vi "rad_Deploy Images with Progress.vi"(6 "Deployment Notifiers":T1[](array[typedef]), 7 "temp folder":path, 8 "error in (no error)":errorcluster, 9 "Target Config Options in":T4={"NumInBatch"=0, "Target Config Operation"=enum."No Config", "Target Name"="", "Increment Static IPs"=FALSE, "Change Target Name"=FALSE, "Primary NIC"={"MAC address"="", "IP Address Request Mode"=2, "IP address"="", "Subnet mask"="", "Gateway"="", "DNS server"=""}} {"Primary NIC"."IP Address Request Mode" items=["Static"=1, "DHCP/Link-Local"=2, "Link-Local Only"=4, "DHCP Only"=8]}, 10 "RT Deployment Targets in":T2[](array[typedef]) {"Primary NIC"."IP Address Request Mode" items=["Static"=1, "DHCP/Link-Local"=2, "Link-Local Only"=4, "DHCP Only"=8]}, 11 "image path":path) -> (0 "error out":errorcluster, 1 "Target Config Options out":T4={"NumInBatch"=0, "Target Config Operation"=enum."No Config", "Target Name"="", "Increment Static IPs"=FALSE, "Change Target Name"=FALSE, "Primary NIC"={"MAC address"="", "IP Address Request Mode"=2, "IP address"="", "Subnet mask"="", "Gateway"="", "DNS server"=""}} {"Primary NIC"."IP Address Request Mode" items=["Static"=1, "DHCP/Link-Local"=2, "Link-Local Only"=4, "DHCP Only"=8]}, 2 "Error Occurred":bool[](array[boolean]))   [LabVIEW 2013]
uses:
  TypeDefs/rad_Target Configuration Settings.ctl
  TypeDefs/rad_Target Configuration Operations.ctl
  Targets/TypeDefs/rad_Target Network Settings.ctl
  Targets/TypeDefs/rad_Target Information.ctl
  TypeDefs/rad_Application Image Properties.ctl
  TypeDefs/rad_FPGA Properties.ctl
  TypeDefs/rad_FPGA Flash Properties.ctl
  TypeDefs/rad_Deployment Notifiers.ctl
  TypeDefs/rad_Deployment Status Data Type.ctl
  TypeDefs/rad_Deployment Progress Data Type.ctl
  Targets/TypeDefs/rad_Initialize Access Types.ctl
  <vilib>/nisyscfg/Close (System).vi
  <vilib>/nisyscfg/Set System Image (Folder).vi
  <vilib>/nisyscfg/nisyscfg.lvlib
panel:
  in  "State Variables":T10={"INI Modified"=FALSE, "Target Config. Options"={"NumInBatch"=0, "Target Config Operation"=enum."No Config", "Target Name"="", "Increment Static IPs"=FALSE, "Change Target Name"=FALSE, "Primary NIC"={"MAC address"="", "IP Address Request Mode"=2, "IP address"="", "Subnet mask"="", "Gateway"="", "DNS server"=""}}, "RT Deployment Targets"=[], "AppImage Properties"={"Name"="", "Version"="", "Time"=timestamp(0 s since 1904-01-01), "Description"="", "Key"="", "Chassis"="", "FPGA Properties"=[], "Model"="", "Retrieve"=[], "Deploy"=[], "Installed Software"=[]}, "Deployment Notifiers"=[], "Post-deployment access"=enum."Admin unless unlocked"} {"RT Deployment Targets"."Primary NIC"."IP Address Request Mode" items=["Static"=1, "DHCP/Link-Local"=2, "Link-Local Only"=4, "DHCP Only"=8]; "Target Config. Options"."Primary NIC"."IP Address Request Mode" items=["Static"=1, "DHCP/Link-Local"=2, "Link-Local Only"=4, "DHCP Only"=8]}
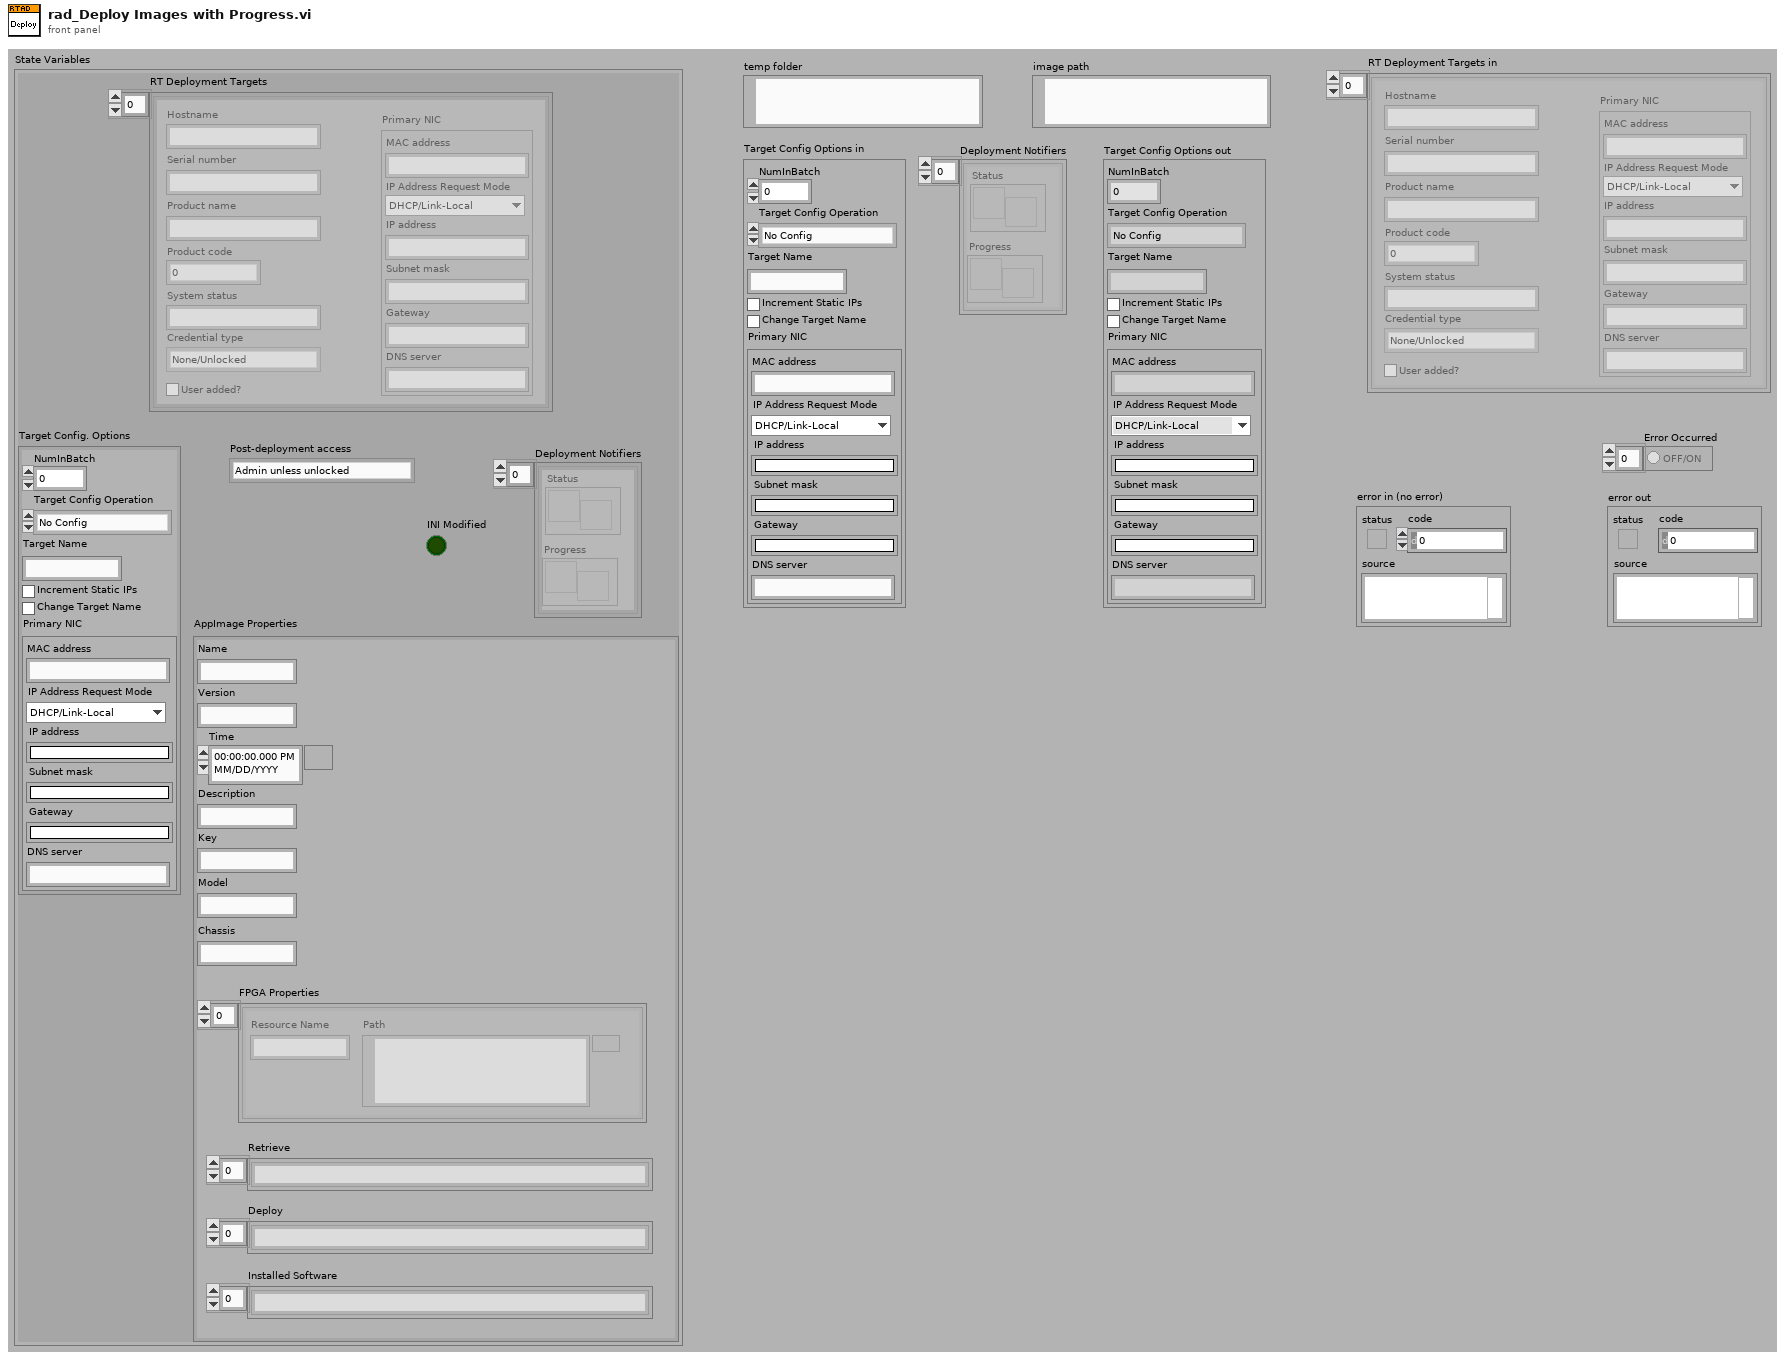
[diagram p1: front panel]
types:
  T1 = typedef "rad_Deployment Notifiers.ctl" = cluster{"Status":refnum<notifier>, "Progress":refnum<notifier>}
  T2 = typedef "rad_Target Information.ctl" = cluster{"Hostname":string, "Serial number":string, "Product name":string, "Product code":i32, "System status":string, "Credential type":enum16{"None/Unlocked", "FTP Password", "NIAuth Credentials"}, "User added?":bool, "Primary NIC":T3}
  T3 = typedef "rad_Target Network Settings.ctl" = cluster{"MAC address":string, "IP Address Request Mode":i32, "IP address":string, "Subnet mask":string, "Gateway":string, "DNS server":string}
  T4 = typedef "rad_Target Configuration Settings.ctl" = cluster{"NumInBatch":u32, "Target Config Operation":T5, "Target Name":string, "Increment Static IPs":bool, "Change Target Name":bool, "Primary NIC":T3}
  T5 = typedef "rad_Target Configuration Operations.ctl" = enum8{"No Config", "Image Config", "Static Config"}
  T6 = typedef "rad_Application Image Properties.ctl" = cluster{"Name":string, "Version":string, "Time":timestamp, "Description":string, "Key":string, "Chassis":string, "FPGA Properties":T7, "Model":string, "Retrieve":string[], "Deploy":string[], "Installed Software":string[]}
  T7 = typedef "rad_FPGA Properties.ctl" = T8[]
  T8 = typedef "rad_FPGA Flash Properties.ctl" = cluster{"Resource Name":string, "Path":path}
  T9 = typedef "rad_Initialize Access Types.ctl" = enum16{"Anonymous read-only", "Admin unless unlocked", "Admin always"}
  T10 = cluster{"INI Modified":bool, "Target Config. Options":T4, "RT Deployment Targets":T2[], "AppImage Properties":T6, "Deployment Notifiers":T1[], "Post-deployment access":T9}
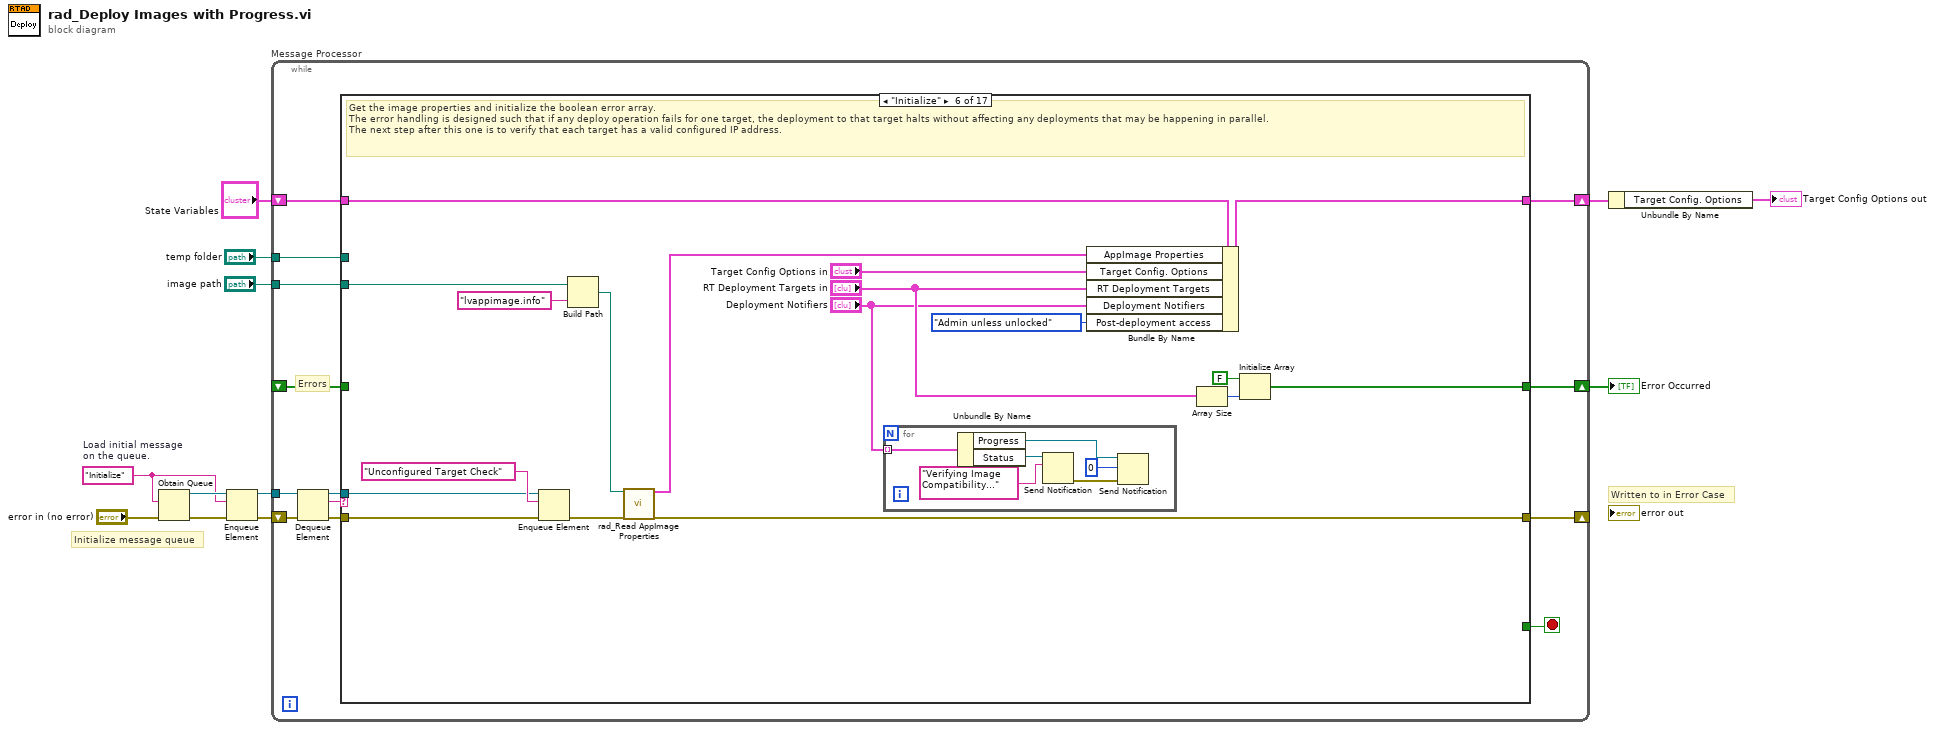
[diagram p0: block diagram]
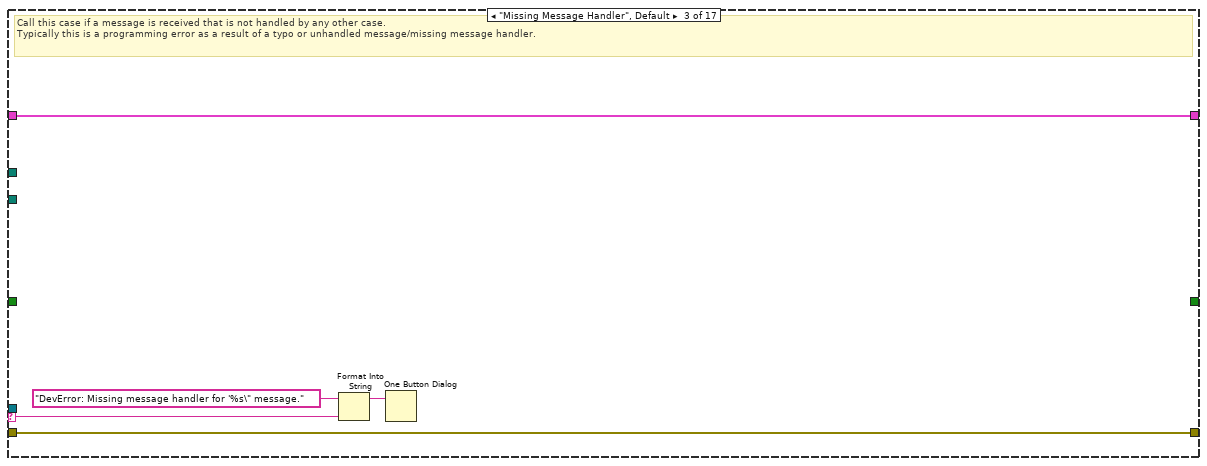
[diagram p4: hidden frame]
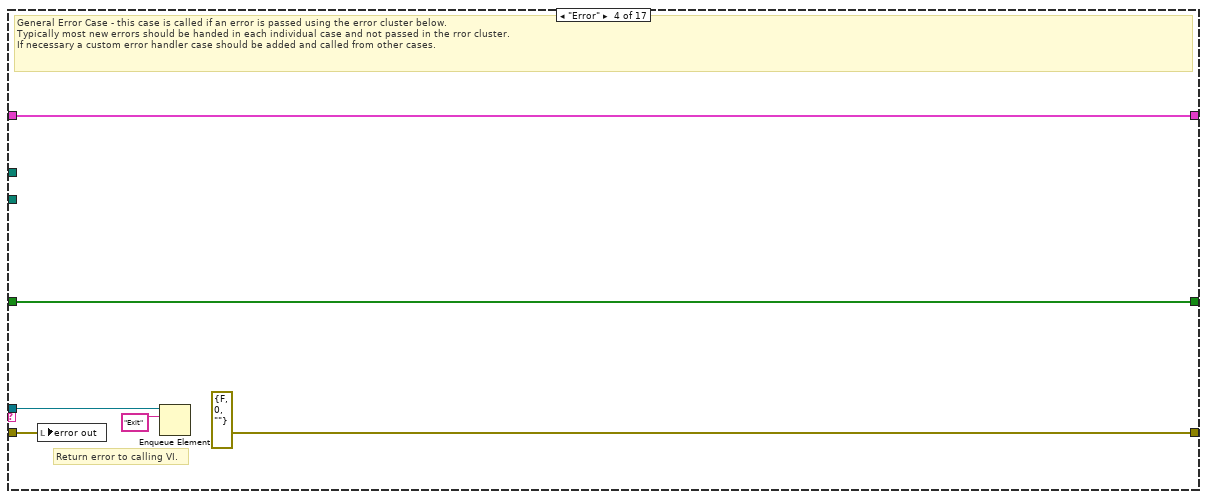
[diagram p5: hidden frame]
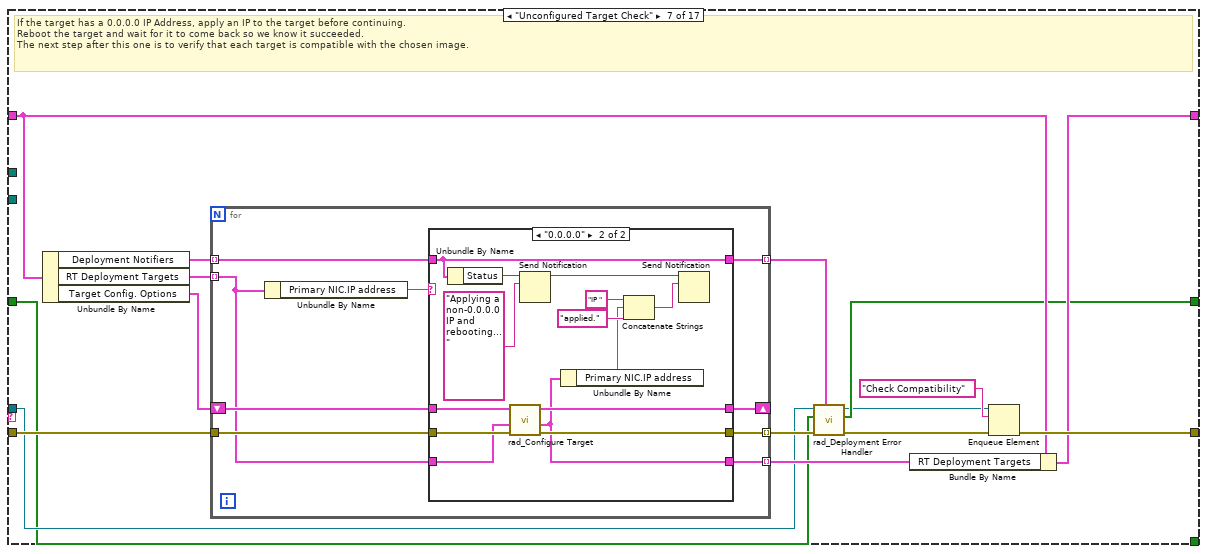
[diagram p7: hidden frame]
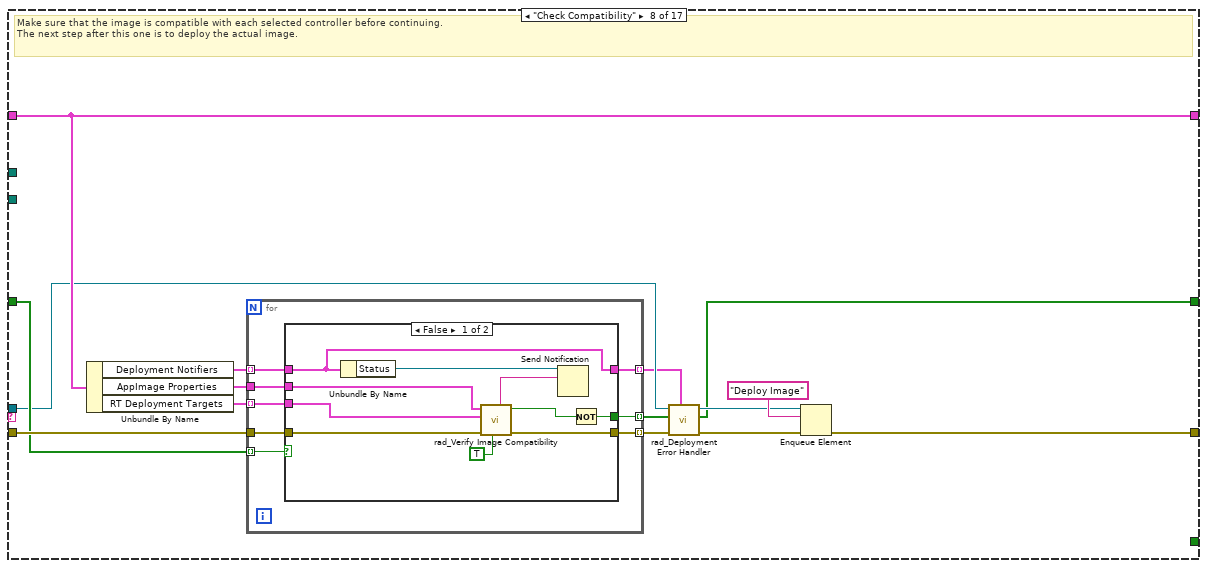
[diagram p9: hidden frame]
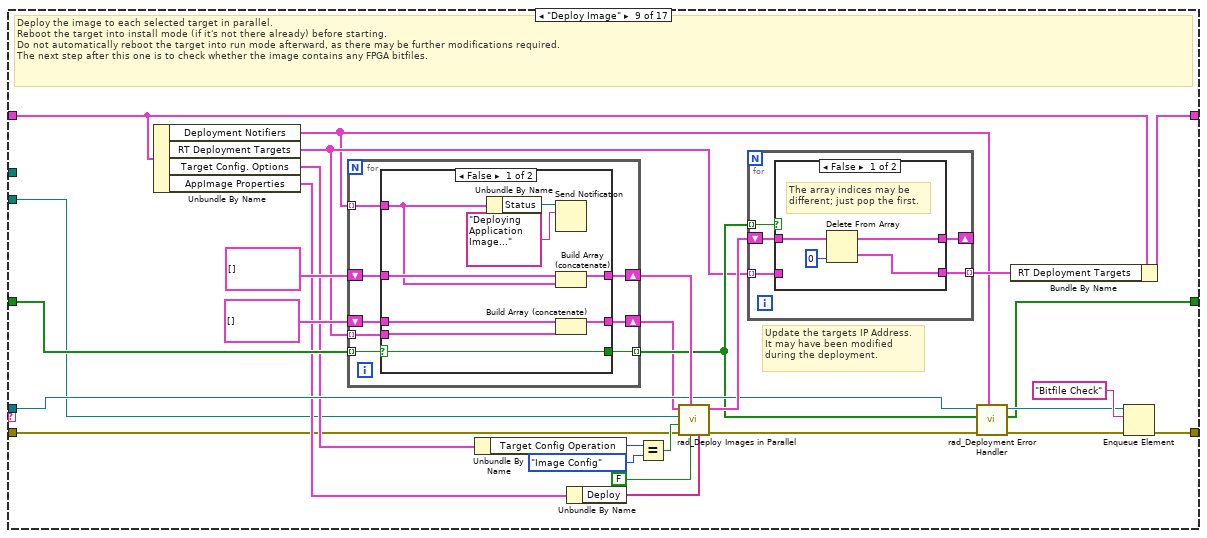
[diagram p11: hidden frame]
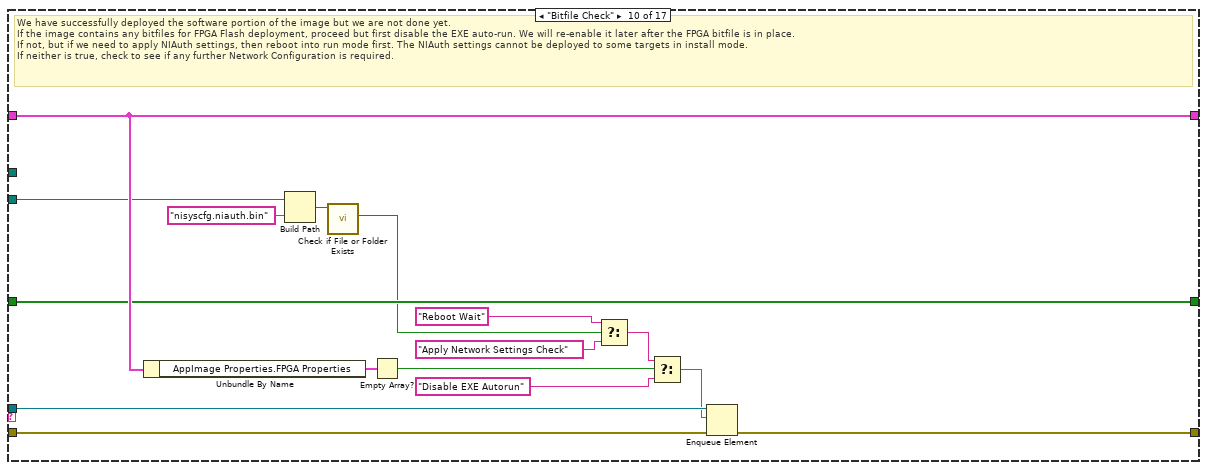
[diagram p14: hidden frame]
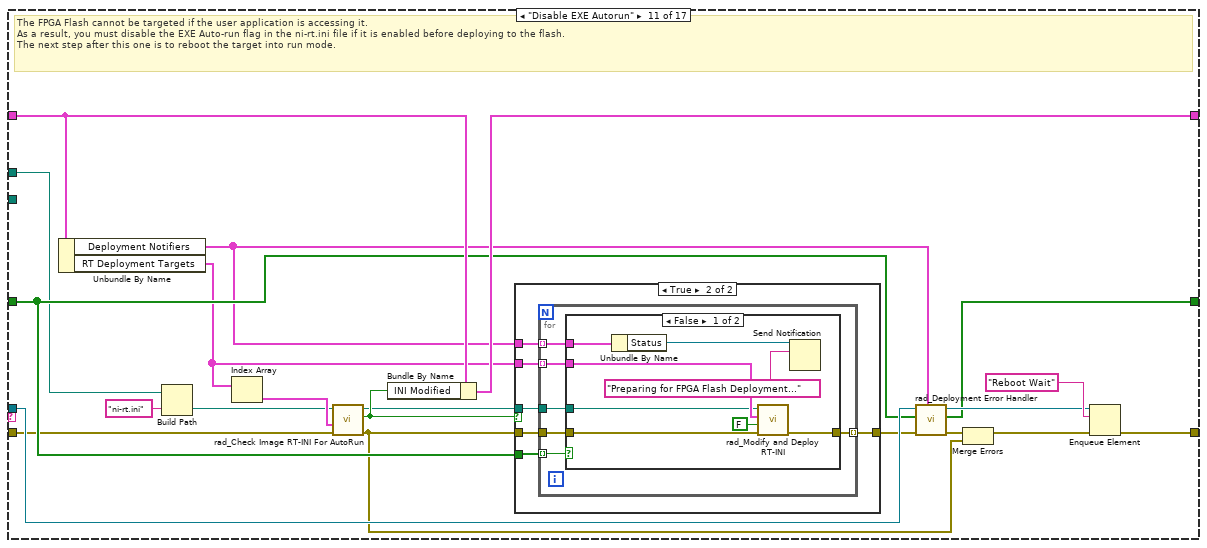
[diagram p15: hidden frame]
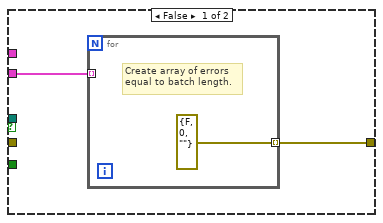
[diagram p16: hidden frame]
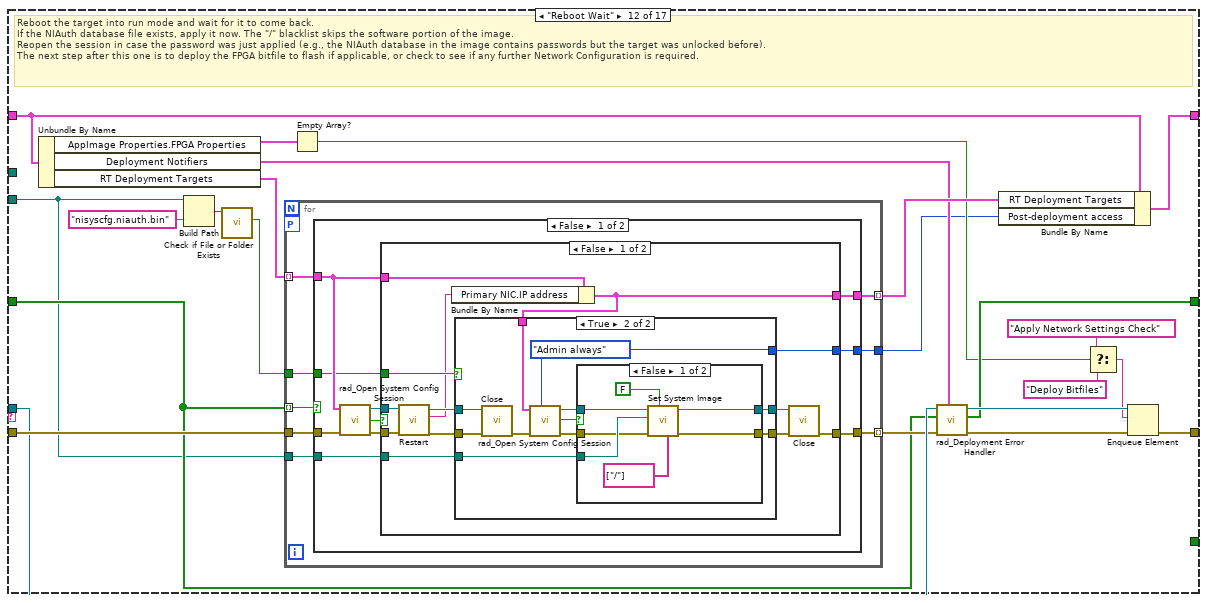
[diagram p18: hidden frame]
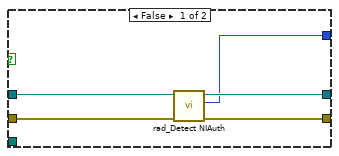
[diagram p19: hidden frame]
diagram:
  w1 = "Initialize"  # Load initial message on the queue.
  # "Written to in Error Case"
  # "Initialize message queue"
  n1 = Obtain Queue(element data type=w1, error in (no error)="error in (no error)") -> (queue out=w12:refnum<queue>, error out=w3:errorcluster)  [unwired: 3 in, 1 out]
  n2 = Enqueue Element(queue=w12, element=w1, error in (no error)=w3) -> (queue out=w4:refnum<queue>, error out=w2:errorcluster)  [unwired: 1 in, 1 out]
  n3 = while "Message Processor" {
    shift-left: w2 -> [w21]
    shift-right: [w14] -> _
    tunnel: w4 -> [w22]
    shift-left: "State Variables" -> [w25]
    shift-right: [w24] -> w9
    tunnel: "temp folder" -> [w18]
    tunnel: "image path" -> [w17]
    shift-right: [w15] -> w5
    shift-left: _ -> [w16]
    stop <- w13 stop-if-true
    # "Errors"
    n4 = Dequeue Element(queue=w22, error in (no error)=w21) -> (queue out=w23:refnum<queue>, element=w19:string, error out=w20:errorcluster)  [unwired: 1 in, 1 out]
    n5 = case shown="\"Initialize\"" w19 {
      selector: w19 -> [_ _ w33 _ _ _ _ _ _ _ _ _ _ _ _ _ _]
      tunnel: [w27 w30 w35 w41 w43 w60 w80 w124 w166 w219 w239 w284 w372 w412 w441 w488 w512] -> w24
      tunnel: w25 -> [w27 w30 w35 w41 w43 w61 w79 w124 w167 w219 w240 w286 w372 w412 w439 w488 w512]
      tunnel: w23 -> [_ _ _ w40 _ w45 w70 w117 w164 w220 w238 w282 w366 w409 w432 w495 w514]
      tunnel: w20 -> [w26 w29 w34 w37 w42 w50 w83 w119 w147 w218 w224 w287 w355 w400 w440 w497 w515]
      tunnel: [w26 w29 w34 errorcluster {"status"=FALSE, "code"=0, "source"=""} ("error out") w42 w51 w82 w125 w174 w221 w242 w289 w373 w411 w445 w499 w513] -> w14
      tunnel: w18 -> [_ _ _ _ _ _ _ _ _ _ w225 _ _ w401 _ _ _]
      tunnel: w17 -> [_ _ _ _ _ w49 _ _ w148 w213 _ w272 w354 _ _ _ _]
      tunnel: [_ w28 _ w36 _ w56 w74 w112 w159 w217 w235 w280 w365 w407 w430 w493 w510] -> w15
      tunnel: w16 -> [_ w28 _ w36 _ _ w68 w118 w172 w217 w232 w277 w361 w405 w425 w490 w510]
      tunnel: [_ _ _ _ _ _ _ _ _ _ _ _ _ _ _ _ TRUE] -> w13
      frame "---------- Framework Operations ----------" {
        # "Dummy case to add a seperator in the Case Structure menu."
      }
      frame "", "Idle" {
        # "Idle Case - this case is called after a Timeout on the Get Next Message from Queue VI, if no new messages are present on the queue.\nThis case can be used for housekeeping tasks such as updating the UI."
      }
      frame "Missing Message Handler", Default {
        # "Call this case if a message is received that is not handled by any other case.\nTypically this is a programming error as a result of a typo or unhandled message/missing message handler."
        n6 = Format Into String(format string="DevError: Missing message handler for '%s\" message." ("message"), w33) -> (resulting string=w31:string)  [unwired: 2 in, 1 out]
        n7 = One Button Dialog(message=w31) -> ()  [unwired: 2 out]
      }
      frame "Error" {
        # "Return error to calling VI."
        # "General Error Case - this case is called if an error is passed using the error cluster below.\nTypically most new errors should be handed in each individual case and not passed in the rror cluster.\nIf necessary a custom error handler case should be added and called from other cases."
        n8 = local write "error out"(w37) -> ()
        n9 = Enqueue Element(queue=w40, element="Exit") -> ()  [unwired: 2 in, 3 out]
      }
      frame "----------Application Operations ----------" {
        # "Dummy case to add a seperator in the Case Structure menu."
      }
      frame "Initialize" {
        # "Get the image properties and initialize the boolean error array. \nThe error handling is designed such that if any deploy operation fails for one target, the deployment to that target halts without affecting any deployments that may be happening in parallel. \nThe next step after this one is to verify that each target has a valid configured IP address."
        n10 = Enqueue Element(queue=w45, element="Unconfigured Target Check", error in (no error)=w50) -> (error out=w47:errorcluster)  [unwired: 1 in, 2 out]
        n11 = Build Path(base path=w49, name or relative path="lvappimage.info") -> (appended path=w52:path)
        n12 = call "rad_Read AppImage Properties.vi"("AppImage Properties Path"=w52, "error in (no error)"=w47) -> ("AppImage Properties"=w48:T6, "error out"=w51:errorcluster)  [unwired: 12 in, 4 out]
        n13 = for {
          tunnel: "Deployment Notifiers" -> [w66] mode=indexing
          n14 = Unbundle By Name(w66) -> ("Progress"=w64:refnum<notifier>, "Status"=w65:refnum<notifier>)
          n15 = Send Notification(notification="Verifying Image Compatibility...", notifier=w65) -> (error out=w63:errorcluster)  [unwired: 1 in, 1 out]
          n16 = Send Notification(notification=0, notifier=w64, error in (no error)=w63) -> ()  [unwired: 2 out]
        }
        n17 = Bundle By Name(cluster=w61, "AppImage Properties"=w48, "Target Config. Options"="Target Config Options in", "RT Deployment Targets"="RT Deployment Targets in", "Deployment Notifiers"="Deployment Notifiers", "Post-deployment access"=rad_Initialize_Access_Types."Admin unless unlocked") -> (w60:T10)
        n18 = Array Size(array="RT Deployment Targets in") -> (size(s)=w57:i32)
        n19 = Initialize Array(FALSE, w57) -> (w56:bool[])
      }
      frame "Unconfigured Target Check" {
        # "If the target has a 0.0.0.0 IP Address, apply an IP to the target before continuing. \nReboot the target and wait for it to come back so we know it succeeded. \nThe next step after this one is to verify that each target is compatible with the chosen image."
        n20 = Unbundle By Name(w79) -> ("Deployment Notifiers"=w78:T1[], "RT Deployment Targets"=w77:T2[], "Target Config. Options"=w76:T4)
        n21 = for {
          tunnel: w83 -> [w90]
          tunnel: [w92] -> w73 mode=indexing
          tunnel: w78 -> [w88] mode=indexing
          tunnel: w77 -> [w87] mode=indexing
          shift-right: [w89] -> _
          shift-left: w76 -> [w91]
          tunnel: [w86] -> w75 mode=indexing
          tunnel: [w85] -> w71 mode=indexing
          n22 = Unbundle By Name(w87) -> ("Primary NIC.IP address"=w84:string)
          n23 = case shown="\"0.0.0.0\"" w84 {
            tunnel: [w96 w102] -> w92
            tunnel: w91 -> [w94 w110]
            tunnel: w90 -> [w96 w103]
            tunnel: [w94 w109] -> w89
            tunnel: w88 -> [w93 w100]
            tunnel: w87 -> [w95 w99]
            tunnel: [w95 w98] -> w86
            tunnel: [w93 w100] -> w85
            frame Default {
            }
            frame "0.0.0.0" {
              n24 = Unbundle By Name(w100) -> ("Status"=w101:refnum<notifier>)
              n25 = call "rad_Configure Target.vi"("error in (no error)"=w103, "Target settings in"=w99, "Target Config Options in"=w110) -> ("error out"=w102:errorcluster, "Target settings out"=w98:T2, "Target Config Options out"=w109:T4)  [unwired: 6 in]
              n26 = Send Notification(notification="Applying a non-0.0.0.0 IP and rebooting...", notifier=w101) -> (notifier out=w107:refnum<notifier>)  [unwired: 1 in, 1 out]
              n27 = Unbundle By Name(w98) -> ("Primary NIC.IP address"=w97:string)
              n28 = Concatenate Strings("IP " ("notification"), w97, "applied." ("string")) -> (w104:string)
              n29 = Send Notification(notification=w104, notifier=w107) -> ()  [unwired: 1 in, 2 out]
            }
          }
        }
        n30 = call "rad_Deployment Error Handler.vi"("Deployment Notifiers"=w71, "error in (no error)"=w73, "Error Occurred"=w68, "Queue in"=w70) -> ("error out"=w72:errorcluster, "Error Occurred"=w74:bool[], "Queue out"=w69:refnum<queue>)  [unwired: 5 in]
        n31 = Bundle By Name(cluster=w79, "RT Deployment Targets"=w75) -> (w80:T10)
        n32 = Enqueue Element(queue=w69, element="Check Compatibility" ("Message Name"), error in (no error)=w72) -> (error out=w82:errorcluster)  [unwired: 1 in, 2 out]
      }
      frame "Check Compatibility" {
        # "Make sure that the image is compatible with each selected controller before continuing.\nThe next step after this one is to deploy the actual image."
        n33 = Unbundle By Name(w124) -> ("Deployment Notifiers"=w121:T1[], "AppImage Properties"=w120:T6, "RT Deployment Targets"=w122:T2[])
        n34 = for {
          tunnel: w122 -> [w131] mode=indexing
          tunnel: w121 -> [w129] mode=indexing
          tunnel: w120 -> [w133]
          tunnel: w119 -> [w132]
          tunnel: w118 -> [w130] mode=indexing
          tunnel: [w128] -> w115 mode=indexing
          tunnel: [w127] -> w116 mode=indexing
          tunnel: [w126] -> w114 mode=indexing
          n35 = case shown="False" w130 {
            selector: w130 -> [_ w146]
            tunnel: w133 -> [w143 _]
            tunnel: w132 -> [w142 w145]
            tunnel: w131 -> [w134 _]
            tunnel: w129 -> [w136 w144]
            tunnel: [w138 w146] -> w128
            tunnel: [w140 w145] -> w127
            tunnel: [w136 w144] -> w126
            frame False {
              n36 = Unbundle By Name(w136) -> ("Status"=w137:refnum<notifier>)
              n37 = call "rad_Verify Image Compatibility.vi"("Require Identical Chassis?"=TRUE, "error in (no error)"=w142, "Target address"=w134, "AppImage Properties"=w143) -> ("error out"=w140:errorcluster, "Compatible?"=w139:bool, "Status message"=w135:string)  [unwired: 5 in]
              n38 = Send Notification(notification=w135, notifier=w137) -> ()  [unwired: 1 in, 2 out]
              n39 = Not(x=w139) -> (.not. x?=w138:bool)
            }
            frame True {
            }
          }
        }
        n40 = call "rad_Deployment Error Handler.vi"("Deployment Notifiers"=w114, "error in (no error)"=w116, "Error Occurred"=w115, "Queue in"=w117) -> ("error out"=w111:errorcluster, "Error Occurred"=w112:bool[], "Queue out"=w113:refnum<queue>)  [unwired: 5 in]
        n41 = Enqueue Element(queue=w113, element="Deploy Image" ("t"), error in (no error)=w111) -> (error out=w125:errorcluster)  [unwired: 1 in, 2 out]
      }
      frame "Deploy Image" {
        # "Update the targets IP Address.\nIt may have been modified\nduring the deployment."
        # "Deploy the image to each selected target in parallel. \nReboot the target into install mode (if it's not there already) before starting.\nDo not automatically reboot the target into run mode afterward, as there may be further modifications required. \nThe next step after this one is to check whether the image contains any FPGA bitfiles."
        n42 = Unbundle By Name(w167) -> ("Deployment Notifiers"=w156:T1[], "RT Deployment Targets"=w157:T2[], "Target Config. Options"=w152:T4, "AppImage Properties"=w151:T6)
        n43 = for {
          tunnel: w156 -> [w192] mode=indexing
          tunnel: w172 -> [w193] mode=indexing
          tunnel: [w191] -> w162 mode=indexing
          tunnel: w157 -> [w190] mode=indexing
          shift-right: [w189] -> w169
          shift-left: T1[] [] ("Deployment Notifiers") -> [w188]
          shift-right: [w187] -> w149
          shift-left: T2[] [] -> [w186]
          n44 = case shown="False" w193 {
            selector: w193 -> [w201 w205]
            tunnel: w192 -> [w196 _]
            tunnel: [w201 w205] -> w191
            tunnel: w190 -> [w194 _]
            tunnel: [w200 w203] -> w189
            tunnel: w188 -> [w199 w203]
            tunnel: [w198 w204] -> w187
            tunnel: w186 -> [w197 w204]
            frame False {
              n45 = Unbundle By Name(w196) -> ("Status"=w195:refnum<notifier>)
              n46 = Send Notification(notification="Deploying Application Image...", notifier=w195) -> ()  [unwired: 1 in, 2 out]
              n47 = Build Array (concatenate)(w199, w196) -> (w200:T1[])
              n48 = Build Array (concatenate)(w197, w194) -> (w198:T2[])
            }
            frame True {
            }
          }
        }
        n49 = Unbundle By Name(w152) -> ("Target Config Operation"=w155:T5)
        n50 = Unbundle By Name(w151) -> ("Deploy"=w150:string[])
        n51 = Equal?(x=w155, y=rad_Target_Configuration_Operations."Image Config" ("x")) -> (x = y?=w153:bool)
        n52 = call "rad_Deploy Images in Parallel.vi"("Deploy"=w150, "restart after imaging (T)"=FALSE ("restart after imaging? (T)"), "Deployment Notifiers"=w169, "error in (no error)"=w147, "apply primary NIC from image (F)"=w153, "image file path in"=w148, "Target addresses in"=w149) -> ("Errors Out"=w163:errorcluster[], "Target addresses out"=w168:T2[])  [unwired: 2 in, 1 out]
        n53 = for {
          tunnel: w162 -> [w179] mode=indexing
          tunnel: w157 -> [w177] mode=indexing
          shift-right: [w175] -> _
          shift-left: w168 -> [w178]
          tunnel: [w176] -> w165 mode=indexing
          n54 = case shown="False" w179 {
            tunnel: w178 -> [w183 w185]
            tunnel: w177 -> [_ w184]
            tunnel: [w181 w184] -> w176
            tunnel: [w182 w185] -> w175
            frame False {
              # "The array indices may be\ndifferent; just pop the first."
              n55 = Delete From Array(array=w183, index=0) -> (deleted portion=w181:T2, array with subset deleted=w182:T2[])  [unwired: 1 in]
            }
            frame True {
              # "An error happened earlier,\nso keep the existing address."
            }
          }
        }
        n56 = call "rad_Deployment Error Handler.vi"("Deployment Notifiers"=w156, "error in (no error)"=w163, "Error Occurred"=w162, "Queue in"=w164) -> ("error out"=w160:errorcluster, "Error Occurred"=w159:bool[], "Queue out"=w161:refnum<queue>)  [unwired: 5 in]
        n57 = Bundle By Name(cluster=w167, "RT Deployment Targets"=w165) -> (w166:T10)
        n58 = Enqueue Element(queue=w161, element="Bitfile Check" ("Message Name"), error in (no error)=w160) -> (error out=w174:errorcluster)  [unwired: 1 in, 2 out]
      }
      frame "Bitfile Check" {
        # "We have successfully deployed the software portion of the image but we are not done yet.\nIf the image contains any bitfiles for FPGA Flash deployment, proceed but first disable the EXE auto-run. We will re-enable it later after the FPGA bitfile is in place.\nIf not, but if we need to apply NIAuth settings, then reboot into run mode first. The NIAuth settings cannot be deployed to some targets in install mode.\nIf neither is true, check to see if any further Network Configuration is required."
        n59 = Unbundle By Name(w219) -> ("AppImage Properties.FPGA Properties"=w216:T7)
        n60 = Build Path(base path=w213, name or relative path="nisyscfg.niauth.bin") -> (appended path=w211:path)
        n61 = call <vilib>:"Check if File or Folder Exists.vi"("path"=w211) -> ("file or folder exists?"=w208:bool)  [unwired: 8 in, 2 out]
        n62 = Empty Array?(array=w216) -> (empty?=w214:bool)
        n63 = Select(t="Reboot Wait" ("Title"), s=w208, f="Apply Network Settings Check" ("Title")) -> (s? t:f=w209:string)
        n64 = Select(t=w209, s=w214, f="Disable EXE Autorun" ("Title")) -> (s? t:f=w210:string)
        n65 = Enqueue Element(queue=w220, element=w210, error in (no error)=w218) -> (error out=w221:errorcluster)  [unwired: 1 in, 2 out]
      }
      frame "Disable EXE Autorun" {
        # "The FPGA Flash cannot be targeted if the user application is accessing it.\nAs a result, you must disable the EXE Auto-run flag in the ni-rt.ini file if it is enabled before deploying to the flash.\nThe next step after this one is to reboot the target into run mode."
        n66 = Unbundle By Name(w240) -> ("Deployment Notifiers"=w231:T1[], "RT Deployment Targets"=w230:T2[])
        n67 = Build Path(base path=w225, name or relative path="ni-rt.ini") -> (appended path=w223:path)
        n68 = Index Array(array=w230) -> (element=w226:T2)  [unwired: 1 in]
        n69 = call "rad_Check Image RT-INI For AutoRun.vi"("error in (no error)"=w224, "target settings"=w226, "temp folder"=w223) -> ("error out"=w229:errorcluster, "Run at Startup?"=w228:bool, "temp folder out"=w227:path)  [unwired: 6 in]
        n70 = Bundle By Name(cluster=w240, "INI Modified"=w228) -> (w239:T10)
        n71 = case shown="True" w228 {
          tunnel: [w243 w250] -> w236
          tunnel: w229 -> [_ w251]
          tunnel: w230 -> [w244 w249]
          tunnel: w232 -> [_ w248]
          tunnel: w231 -> [_ w247]
          tunnel: w227 -> [_ w246]
          frame False {
            n72 = for {
              tunnel: w244 -> [_] mode=indexing
              tunnel: [errorcluster {"status"=FALSE, "code"=0, "source"=""} ("error out")] -> w243 mode=indexing
              # "Create array of errors\nequal to batch length."
            }
          }
          frame True {
            n73 = for {
              tunnel: w251 -> [w257]
              tunnel: [w256] -> w250 mode=indexing
              tunnel: w249 -> [w255] mode=indexing
              tunnel: w248 -> [w254] mode=indexing
              tunnel: w247 -> [w253] mode=indexing
              tunnel: w246 -> [w252]
              n74 = case shown="False" w254 {
                tunnel: w257 -> [w259 w266]
                tunnel: [w264 w266] -> w256
                tunnel: w255 -> [w260 _]
                tunnel: w253 -> [w262 _]
                tunnel: w252 -> [w258 _]
                frame False {
                  n75 = Unbundle By Name(w262) -> ("Status"=w261:refnum<notifier>)
                  n76 = call "rad_Modify and Deploy RT-INI.vi"("error in (no error)"=w259, "Run at Startup?"=FALSE, "Target settings"=w260, "temp folder"=w258) -> ("error out"=w264:errorcluster)  [unwired: 7 in]
                  n77 = Send Notification(notification="Preparing for FPGA Flash Deployment...", notifier=w261) -> ()  [unwired: 1 in, 2 out]
                }
                frame True {
                }
              }
            }
          }
        }
        n78 = call "rad_Deployment Error Handler.vi"("Deployment Notifiers"=w231, "error in (no error)"=w236, "Error Occurred"=w232, "Queue in"=w238) -> ("error out"=w234:errorcluster, "Error Occurred"=w235:bool[], "Queue out"=w237:refnum<queue>)  [unwired: 5 in]
        n79 = Merge Errors(w234, w229) -> (w233:errorcluster)
        n80 = Enqueue Element(queue=w237, element="Reboot Wait" ("Message Name"), error in (no error)=w233) -> (error out=w242:errorcluster)  [unwired: 1 in, 2 out]
      }
      frame "Reboot Wait" {
        # "Reboot the target into run mode and wait for it to come back.\nIf the NIAuth database file exists, apply it now. The \"/\" blacklist skips the software portion of the image.\nReopen the session in case the password was just applied (e.g., the NIAuth database in the image contains passwords but the target was unlocked before).\nThe next step after this one is to deploy the FPGA bitfile to flash if applicable, or check to see if any further Network Configuration is required."
        n81 = Unbundle By Name(w286) -> ("AppImage Properties.FPGA Properties"=w276:T7, "Deployment Notifiers"=w283:T1[], "RT Deployment Targets"=w288:T2[])
        n82 = Build Path(base path=w272, name or relative path="nisyscfg.niauth.bin") -> (appended path=w274:path)
        n83 = call <vilib>:"Check if File or Folder Exists.vi"("path"=w274) -> ("file or folder exists?"=w273:bool)  [unwired: 8 in, 2 out]
        n84 = for {
          tunnel: w288 -> [w295] mode=indexing
          tunnel: w287 -> [w297]
          tunnel: [w296] -> w278 mode=indexing
          tunnel: [w294] -> w285 mode=indexing
          tunnel: w277 -> [w293] mode=indexing
          workers-P: _ -> [_]
          tunnel: w273 -> [w292]
          tunnel: w272 -> [w291]
          tunnel: [w290] -> w267
          n85 = case shown="False" w293 {
            tunnel: w297 -> [w307 w350]
            tunnel: [w300 w350] -> w296
            tunnel: w295 -> [w303 w351]
            tunnel: [w302 w351] -> w294
            tunnel: w292 -> [w301 _]
            tunnel: w291 -> [w299 _]
            tunnel: [w298 rad_Initialize_Access_Types."Admin unless unlocked" ("Access requirement (admin unless unlocked)")] -> w290
            frame False {
              n86 = call "rad_Open System Config Session.vi"("error in (no error)"=w307, "Target settings"=w303) -> ("error out"=w304:errorcluster, "Cancelled"=w306:bool, "Session out"=w305:refnum<k21>)  [unwired: 6 in, 1 out]
              n87 = case shown="False" w306 {
                tunnel: w305 -> [w319 _]
                tunnel: w304 -> [w320 w347]
                tunnel: w303 -> [w311 w348]
                tunnel: [w309 w348] -> w302
                tunnel: w301 -> [w318 _]
                tunnel: [w313 w347] -> w300
                tunnel: w299 -> [w312 _]
                tunnel: [w308 rad_Initialize_Access_Types."Admin unless unlocked" ("Access requirement (admin unless unlocked)")] -> w298
                frame False {
                  n88 = call <vilib>:"Restart.vi"("error in (no error)"=w320, "Session in"=w319) -> ("error out"=w316:errorcluster, "New IP Address"=w310:string, "Session out"=w317:refnum<k21>)  [unwired: 7 in]
                  n89 = Bundle By Name(cluster=w311, "Primary NIC.IP address"=w310) -> (w309:T2)
                  n90 = case shown="True" w318 {
                    tunnel: w317 -> [w325 w332]
                    tunnel: w316 -> [w324 w333]
                    tunnel: [w322 w335] -> w315
                    tunnel: [w323 w336] -> w314
                    tunnel: w312 -> [_ w334]
                    tunnel: [w321 w327] -> w308
                    tunnel: w309 -> [_ w326]
                    frame False {
                      n91 = call "rad_Detect NIAuth.vi"("error in (no error)"=w324, "Session in"=w325) -> ("error out"=w323:errorcluster, "Post-deployment access"=w321:T9, "Session out"=w322:refnum<k21>)  [unwired: 7 in]
                    }
                    frame True {
                      w327 = rad_Initialize_Access_Types."Admin always" ("Access requirement (admin unless unlocked)")
                      n92 = call-poly <vilib>:"Close.vi"("error in (no error)"=w333, "Session in"=w332) -> ("error out"=w331:errorcluster)  [unwired: 9 in]
                      n93 = call "rad_Open System Config Session.vi"("Access requirement (admin unless unlocked)"=w327, "error in (no error)"=w331, "Target settings"=w326) -> ("error out"=w328:errorcluster, "Cancelled"=w330:bool, "Session out"=w329:refnum<k21>)  [unwired: 5 in, 1 out]
                      n94 = case shown="False" w330 {
                        tunnel: [w343 w344] -> w336
                        tunnel: [w342 w345] -> w335
                        tunnel: w334 -> [w339 _]
                        tunnel: w329 -> [w338 w345]
                        tunnel: w328 -> [w337 w344]
                        frame False {
                          n95 = call-poly <vilib>:"Set System Image.vi"("File and Directory Blacklist"=string[] ["/"], "Restart Automatically (T)"=FALSE ("restart automatically (T)"), "error in (no error)"=w337, "Source Folder"=w339, "Session in"=w338) -> ("error out"=w343:errorcluster, "Session out"=w342:refnum<k21>)  [unwired: 5 in]
                        }
                        frame True {
                        }
                      }
                    }
                  }
                  n96 = call-poly <vilib>:"Close.vi"("error in (no error)"=w314, "Session in"=w315) -> ("error out"=w313:errorcluster)  [unwired: 9 in]
                }
                frame True {
                }
              }
            }
            frame True {
            }
          }
        }
        n97 = Empty Array?(array=w276) -> (empty?=w268:bool)
        n98 = call "rad_Deployment Error Handler.vi"("Deployment Notifiers"=w283, "error in (no error)"=w278, "Error Occurred"=w277, "Queue in"=w282) -> ("error out"=w279:errorcluster, "Error Occurred"=w280:bool[], "Queue out"=w281:refnum<queue>)  [unwired: 5 in]
        n99 = Bundle By Name(cluster=w286, "RT Deployment Targets"=w285, "Post-deployment access"=w267) -> (w284:T10)
        n100 = Select(t="Apply Network Settings Check" ("Message Name"), s=w268, f="Deploy Bitfiles" ("Message Name")) -> (s? t:f=w269:string)
        n101 = Enqueue Element(queue=w281, element=w269, error in (no error)=w279) -> (error out=w289:errorcluster)  [unwired: 1 in, 2 out]
      }
      frame "Deploy Bitfiles" {
        # "We have at least one FPGA bitfile and the EXE is not running, so deploy the bitfile to flash now.\nThe next step after this one is to re-enable the EXE Autorun flag in the ni-rt.ini file if it was modified, or check to see if any further Network Configuration is required."
        n102 = Unbundle By Name(w372) -> ("Deployment Notifiers"=w353:T1[], "Post-deployment access"=w352:T9, "RT Deployment Targets"=w367:T2[], "AppImage Properties.FPGA Properties"=w359:T7, "INI Modified"=w368:bool)
        n103 = List Folder(path=w354, pattern="*.lvbitx", error in=w355) -> (filenames=w357:string[])  [unwired: 1 in, 3 out]
        n104 = for {
          tunnel: w354 -> [w376]
          tunnel: w357 -> [w375] mode=indexing
          tunnel: [w374] -> w356 mode=indexing
          n105 = Build Path(base path=w376, name or relative path=w375) -> (appended path=w374:path)
        }
        n106 = for {
          tunnel: w359 -> [w384]
          tunnel: w356 -> [w383]
          tunnel: [w382] -> w364 mode=indexing
          tunnel: w367 -> [w381] mode=indexing
          tunnel: w355 -> [w380]
          tunnel: w353 -> [w379] mode=indexing
          tunnel: w361 -> [w378] mode=indexing
          tunnel: w352 -> [w377]
          n107 = case shown="False" w378 {
            tunnel: w384 -> [w395 _]
            tunnel: w383 -> [w394 _]
            tunnel: [w390 errorcluster {"status"=FALSE, "code"=0, "source"=""} ("error out")] -> w382
            tunnel: w381 -> [w386 _]
            tunnel: w380 -> [w393 _]
            tunnel: w379 -> [w388 _]
            tunnel: w377 -> [w385 _]
            frame False {
              n108 = Unbundle By Name(w388) -> ("Status"=w387:refnum<notifier>)
              n109 = Send Notification(notification="Deploying to FPGA Flash...", notifier=w387) -> (notifier out=w391:refnum<notifier>)  [unwired: 1 in, 1 out]
              n110 = call "rad_Deploy All Bitfiles.vi"("Access requirement"=w385, "error in (no error)"=w393, "FPGA Properties"=w395, "Unzipped files"=w394, "Target settings in"=w386) -> ("error out"=w390:errorcluster)  [unwired: 6 in]
              n111 = Send Notification(notification="FPGA Flash Deployed.", notifier=w391, error in (no error)=w390) -> ()  [unwired: 2 out]
            }
            frame True {
            }
          }
        }
        n112 = call "rad_Deployment Error Handler.vi"("Deployment Notifiers"=w353, "error in (no error)"=w364, "Error Occurred"=w361, "Queue in"=w366) -> ("error out"=w363:errorcluster, "Error Occurred"=w365:bool[], "Queue out"=w360:refnum<queue>)  [unwired: 5 in]
        n113 = Select(t="Enable EXE Autorun" ("Title"), s=w368, f="Apply Network Settings Check") -> (s? t:f=w370:string)
        n114 = Merge Errors(w363, w355) -> (w362:errorcluster)
        n115 = Enqueue Element(queue=w360, element=w370, error in (no error)=w362) -> (error out=w373:errorcluster)  [unwired: 1 in, 2 out]
      }
      frame "Enable EXE Autorun" {
        # "Re-enable the startup EXE in the ni-rt.ini file if it was disabled previously.\nThe next step after this one is to check to see if any further Network Configuration is required."
        n116 = Build Path(base path=w401, name or relative path="ni-rt.ini") -> (appended path=w398:path)
        n117 = Unbundle By Name(w412) -> ("Deployment Notifiers"=w399:T1[], "RT Deployment Targets"=w402:T2[])
        n118 = for {
          tunnel: w398 -> [w417]
          tunnel: w400 -> [w416]
          tunnel: w402 -> [w414] mode=indexing
          tunnel: [w415] -> w408 mode=indexing
          tunnel: w405 -> [w413] mode=indexing
          n119 = case shown="False" w413 {
            tunnel: w417 -> [w418 _]
            tunnel: w416 -> [w419 _]
            tunnel: [w421 errorcluster {"status"=FALSE, "code"=0, "source"=""} ("error out")] -> w415
            tunnel: w414 -> [w420 _]
            frame False {
              n120 = call "rad_Modify and Deploy RT-INI.vi"("error in (no error)"=w419, "Run at Startup?"=TRUE, "Target settings"=w420, "temp folder"=w418) -> ("error out"=w421:errorcluster)  [unwired: 7 in]
            }
            frame True {
            }
          }
        }
        n121 = call "rad_Deployment Error Handler.vi"("Deployment Notifiers"=w399, "error in (no error)"=w408, "Error Occurred"=w405, "Queue in"=w409) -> ("error out"=w404:errorcluster, "Error Occurred"=w407:bool[], "Queue out"=w406:refnum<queue>)  [unwired: 5 in]
        n122 = Merge Errors(w404, w400) -> (w403:errorcluster)
        n123 = Enqueue Element(queue=w406, element="Apply Network Settings Check" ("Message Name"), error in (no error)=w403) -> (error out=w411:errorcluster)  [unwired: 1 in, 2 out]
      }
      frame "Apply Network Settings Check" {
        # "If we need to apply static network settings to each target, do so now.\nReboot each target into run mode and wait for it to come back so we know it succeeded.\nOtherwise, reboot each target into run mode but do not bother waiting for it to come back."
        n124 = Unbundle By Name(w439) -> ("Deployment Notifiers"=w427:T1[], "RT Deployment Targets"=w436:T2[], "Target Config. Options"=w437:T4)
        n125 = Unbundle By Name(w437) -> ("Target Config Operation"=w438:T5)
        n126 = Or Array Elements(Boolean array=w425) -> (logical OR=w426:bool)
        n127 = Equal?(x=w438, y=rad_Target_Configuration_Operations."Static Config") -> (x = y?=w442:bool)
        n128 = case shown="True" w442 {
          tunnel: w440 -> [_ w461]
          tunnel: [w448 w460] -> w431
          tunnel: [w452 w459] -> w435
          tunnel: w437 -> [w452 w458]
          tunnel: w436 -> [w451 w457]
          tunnel: [w451 w456] -> w434
          tunnel: w427 -> [w447 w455]
          tunnel: w426 -> [_ w454]
          tunnel: [w447 w453] -> w424
          frame False {
            n129 = Array Size(array=w451) -> (size(s)=w450:i32)
            n130 = Initialize Array(errorcluster {"status"=FALSE, "code"=0, "source"=""} ("error out"), w450) -> (w448:errorcluster[])
          }
          frame True {
            n131 = for {
              tunnel: w461 -> [w470]
              tunnel: [w469] -> w460 mode=indexing
              tunnel: w457 -> [w466] mode=indexing
              shift-right: [w468] -> w459
              shift-left: w458 -> [w467]
              tunnel: [w465] -> w456 mode=indexing
              tunnel: w455 -> [w464] mode=indexing
              tunnel: w454 -> [w463]
              tunnel: [w462] -> w453 mode=indexing
              n132 = case shown="False" w463 {
                tunnel: w470 -> [w479 w487]
                tunnel: [w474 w487] -> w469
                tunnel: [w483 w486] -> w468
                tunnel: w467 -> [w482 w486]
                tunnel: w466 -> [w472 w485]
                tunnel: [w471 w485] -> w465
                tunnel: w464 -> [w473 w484]
                tunnel: [w473 w484] -> w462
                frame False {
                  n133 = Unbundle By Name(w473) -> ("Status"=w480:refnum<notifier>)
                  n134 = Send Notification(notification="Applying deployment network settings...", notifier=w480, error in (no error)=w479) -> (error out=w478:errorcluster)  [unwired: 1 out]
                  n135 = call "rad_Configure Target.vi"("error in (no error)"=w478, "Target settings in"=w472, "Target Config Options in"=w482) -> ("error out"=w475:errorcluster, "Target settings out"=w471:T2, "Target Config Options out"=w483:T4)  [unwired: 6 in]
                  n136 = Unbundle By Name(w473) -> ("Status"=w477:refnum<notifier>)
                  n137 = Send Notification(notification="Network settings applied.", notifier=w477, error in (no error)=w475) -> (error out=w474:errorcluster)  [unwired: 1 out]
                }
                frame True {
                }
              }
            }
          }
        }
        n138 = Bundle By Name(cluster=w439, "RT Deployment Targets"=w434, "Target Config. Options"=w435) -> (w441:T10)
        n139 = call "rad_Deployment Error Handler.vi"("Deployment Notifiers"=w424, "error in (no error)"=w431, "Error Occurred"=w425, "Queue in"=w432) -> ("error out"=w429:errorcluster, "Error Occurred"=w430:bool[], "Queue out"=w428:refnum<queue>)  [unwired: 5 in]
        n140 = Select(t="Exit", s=w442, f="Reboot No Wait") -> (s? t:f=w433:string)
        n141 = Enqueue Element(queue=w428, element=w433, error in (no error)=w429) -> (error out=w445:errorcluster)  [unwired: 1 in, 2 out]
      }
      frame "Reboot No Wait" {
        # "We're done imaging the target, put it back into run mode."
        n142 = Unbundle By Name(w488) -> ("Deployment Notifiers"=w489:T1[], "RT Deployment Targets"=w498:T2[])
        n143 = for {
          tunnel: w498 -> [w501] mode=indexing
          tunnel: w497 -> [w503]
          tunnel: [w502] -> w492 mode=indexing
          tunnel: w490 -> [w500] mode=indexing
          workers-P: _ -> [_]
          n144 = case shown="False" w500 {
            tunnel: w503 -> [w506 w508]
            tunnel: [w505 w508] -> w502
            tunnel: w501 -> [w504 _]
            frame False {
              n145 = call "rad_Reboot (IP) Wrapper.vi"("error in (no error)"=w506, "wait for restart? (F)"=FALSE, "Target settings in"=w504) -> ("error out"=w505:errorcluster)  [unwired: 7 in, 1 out]
            }
            frame True {
            }
          }
        }
        n146 = call "rad_Deployment Error Handler.vi"("Deployment Notifiers"=w489, "error in (no error)"=w492, "Error Occurred"=w490, "Queue in"=w495) -> ("error out"=w491:errorcluster, "Error Occurred"=w493:bool[], "Queue out"=w494:refnum<queue>)  [unwired: 5 in]
        n147 = Enqueue Element(queue=w494, element="Exit" ("Message Name"), error in (no error)=w491) -> (error out=w499:errorcluster)  [unwired: 1 in, 2 out]
      }
      frame "Exit" {
        # "Nothing left to do!"
        n148 = Release Queue(queue=w514, error in (no error)=w515) -> (error out=w513:errorcluster)  [unwired: 1 in, 2 out]
        n149 = Unbundle By Name(w512) -> ("Deployment Notifiers"=w511:T1[])
        n150 = for {
          tunnel: w511 -> [w517] mode=indexing
          tunnel: w510 -> [w516] mode=indexing
          n151 = case shown="False" w516 {
            tunnel: w517 -> [w518 _]
            frame False {
              n152 = Unbundle By Name(w518) -> ("Status"=w519:refnum<notifier>)
              n153 = Send Notification(notification="Deployment Complete!", notifier=w519) -> ()  [unwired: 1 in, 2 out]
            }
            frame True {
            }
          }
        }
      }
    }
  }
  "Error Occurred" <- w5
  n154 = Unbundle By Name(w9) -> ("Target Config. Options"=→"Target Config Options out":T4)
